vi "Create Results.vi"(8 "error in (no error)":errorcluster, 10 "Results":T1[](array[typedef]), 11 "XML Handler in":refnum<class "XML Handler.lvclass">) -> (0 "error out":errorcluster, 3 "XML Handler out":refnum<class "XML Handler.lvclass">)   [LabVIEW 2020, in "XML Handler.lvclass"]
uses:
  XML Handler.lvclass
  Controls/Result Cluster.ctl
  XML Handler.lvclass/XML Handler.ctl
  <vilib>/xml/Close Reference(Node).vi
  <resource>/objmgr/DOMUserDefRef.rc
  <vilib>/xml/NI_XML.lvlib
panel:
  out "Node Name":string
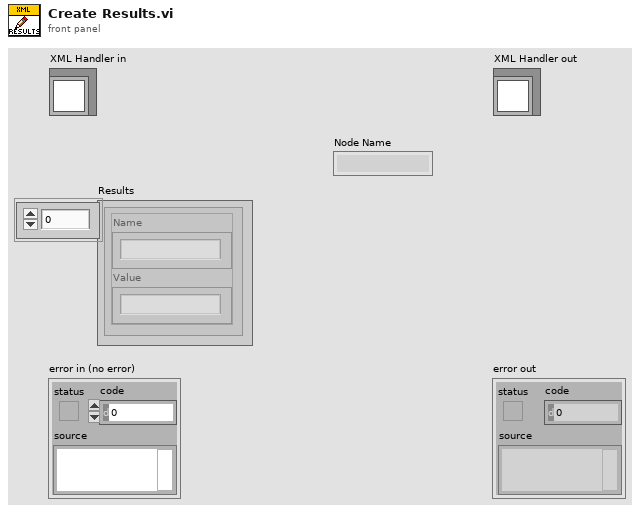
[diagram p1: front panel]
types:
  T1 = typedef "XML Handler.lvclass/Result Cluster.ctl" = cluster{"Name":string, "Value":string}
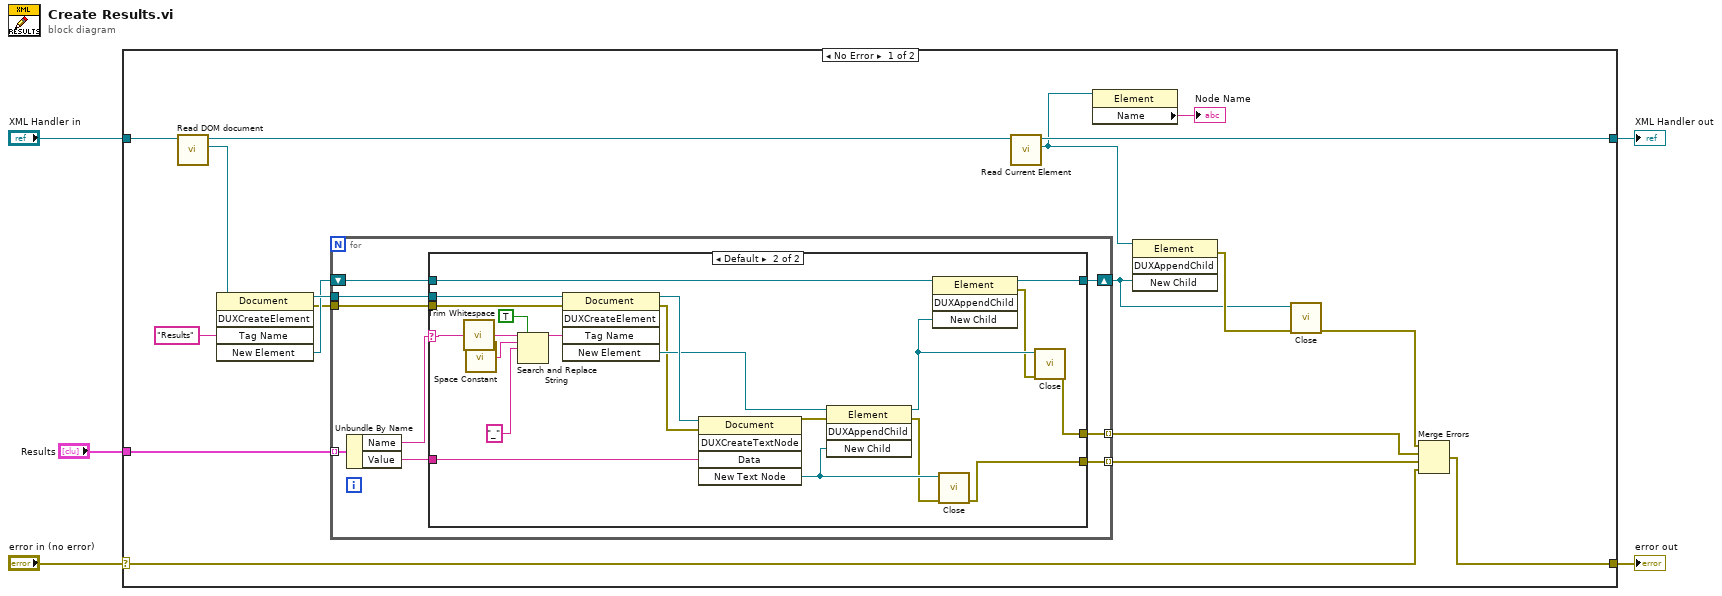
[diagram p0: block diagram]
diagram:
  n1 = case shown="No Error" "error in (no error)" {
    selector: "error in (no error)" -> [w7 w57]
    tunnel: [w6 w57] -> w4
    tunnel: [w20 w56] -> w2
    tunnel: "XML Handler in" -> [w23 w56]
    tunnel: "Results" -> [w21 _]
    frame No Error {
      n2 = call "Read DOM document.vi"("XML Handler in"=w23) -> ("DOM document"=w19:refnum<k20>, "XML Handler out"=w22:refnum<class "XML Handler.lvclass">)  [unwired: 9 in]
      n3 = invoke class="Document" method="DUXCreateElement"(reference=w19, "Tag Name"="Results") -> (reference out=w18:refnum<k20>, error out=w13:errorcluster, "New Element"=w16:refnum<k20>)  [unwired: 3 in, 2 out]
      n4 = for {
        tunnel: w18 -> [w32]
        tunnel: w21 -> [w31] mode=indexing
        tunnel: w13 -> [w27]
        tunnel: [w26] -> w9 mode=indexing
        tunnel: [w25] -> w8 mode=indexing
        shift-right: [w28] -> w14
        shift-left: w16 -> [w29]
        n5 = Unbundle By Name(w31) -> ("Name"=w24:string, "Value"=w30:string)
        n6 = case shown="Default" w24 {
          selector: w24 -> [_ w35]
          tunnel: w32 -> [_ w55]
          tunnel: w30 -> [_ w54]
          tunnel: w29 -> [w34 w47]
          tunnel: [w34 w46] -> w28
          tunnel: w27 -> [w33 w38]
          tunnel: [_ w37] -> w26
          tunnel: [w33 w36] -> w25
          frame "" {
          }
          frame Default {
            n7 = call <vilib>:"Trim Whitespace.vi"("string"=w35) -> ("trimmed string"=w45:string)  [unwired: 1 in]
            n8 = call <vilib>:"Space Constant.vi"() -> ("String"=w43:string)
            n9 = Search and Replace String(replace all?=TRUE ("replace all? (F)"), input string=w45, search string=w43, replace string="_" ("search string")) -> (result string=w44:string)  [unwired: 4 in, 3 out]
            n10 = invoke class="Document" method="DUXCreateElement"(reference=w55, error in=w38, "Tag Name"=w44) -> (reference out=w53:refnum<k20>, error out=w40:errorcluster, "New Element"=w52:refnum<k20>)  [unwired: 2 in, 2 out]
            n11 = invoke class="Document" method="DUXCreateTextNode"(reference=w53, error in=w40, "Data"=w54) -> (error out=w39:errorcluster, "New Text Node"=w51:refnum<k20>)  [unwired: 2 in, 3 out]
            n12 = invoke class="Element" method="DUXAppendChild"(reference=w52, error in=w39, "New Child"=w51) -> (reference out=w49:refnum<k20>, error out=w50:errorcluster)  [unwired: 1 in, 2 out]
            n13 = invoke class="Element" method="DUXAppendChild"(reference=w47, "New Child"=w49) -> (reference out=w46:refnum<k20>, error out=w48:errorcluster)  [unwired: 2 in, 2 out]
            n14 = call-poly <vilib>:"Close.vi"("error in (no error)"=w50, "node"=w51) -> ("error out"=w37:errorcluster)  [unwired: 7 in]
            n15 = call-poly <vilib>:"Close.vi"("error in (no error)"=w48, "node"=w49) -> ("error out"=w36:errorcluster)  [unwired: 7 in]
          }
        }
      }
      n16 = call "Read Current Element.vi"("XML Handler in"=w22) -> ("Current Element"=w12:refnum<k20>, "XML Handler out"=w20:refnum<class "XML Handler.lvclass">)  [unwired: 9 in]
      n17 = property class="Element"(reference=w12) -> ("Name"=→"Node Name":string)  [unwired: 1 in, 2 out]
      n18 = invoke class="Element" method="DUXAppendChild"(reference=w12, "New Child"=w14) -> (error out=w15:errorcluster)  [unwired: 2 in, 3 out]
      n19 = call-poly <vilib>:"Close.vi"("error in (no error)"=w15, "node"=w14) -> ("error out"=w10:errorcluster)  [unwired: 7 in]
      n20 = Merge Errors(w10, w8, w9, w7) -> (w6:errorcluster)
    }
    frame Error {
    }
  }
  "error out" <- w4
  "XML Handler out" <- w2
